vi "temp_probe_initialize.vi"(6 "probe data":string[](array[string]), 8 "error in (no error)":errorcluster, 11 "TempProbe in":refnum<class "TempProbe.lvclass">) -> (0 "error out":errorcluster, 3 "TempProbe out":refnum<class "TempProbe.lvclass">)   [LabVIEW 2010, in "TempProbe.lvclass"]
uses:
  TempProbe.lvclass
  TempProbe.lvclass/TempProbe.ctl
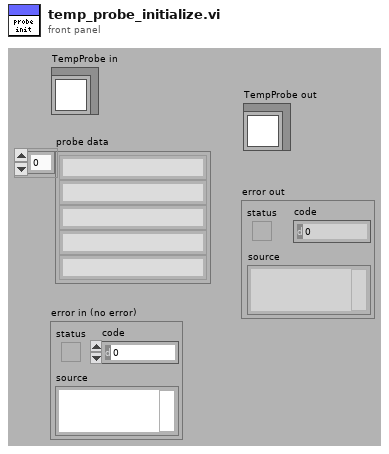
[diagram p1: front panel]
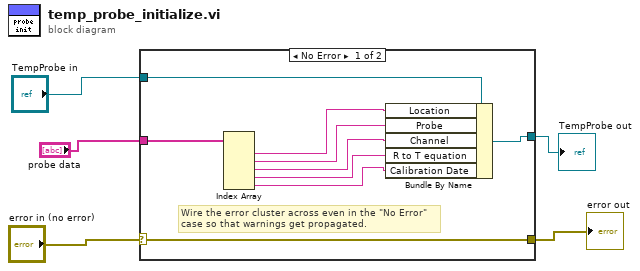
[diagram p0: block diagram]
diagram:
  n1 = case shown="No Error" "error in (no error)" {
    selector: "error in (no error)" -> [w14 w16]
    tunnel: [w14 w16] -> w1
    tunnel: [w12 w15] -> w2
    tunnel: "TempProbe in" -> [w13 w15]
    tunnel: "probe data" -> [w11 _]
    frame No Error {
      # "Wire the error cluster across even in the \"No Error\"\ncase so that warnings get propagated."
      n2 = Index Array(array=w11) -> (element #1=w10:string, element #2=w9:string, element #3=w8:string, element #4=w7:string, element #5=w6:string)  [unwired: 5 in]
      n3 = Bundle By Name(cluster=w13, "Location"=w10, "Probe"=w9, "Channel"=w8, "R to T equation"=w7, "Calibration Date"=w6) -> (w12:refnum<class "TempProbe.lvclass">)
    }
    frame Error {
    }
  }
  "TempProbe out" <- w2
  "error out" <- w1
